vi "shutter_init.vi"(7 "servo":i32(ring)=1 items=["ServoUnspecified", "ServoCh1", "ServoCh2", "ServoBoth"], 8 "error in (no error)":errorcluster, 11 "channel":refnum<k24>) -> (0 "error out":errorcluster)   [LabVIEW 2021]
uses:
  D:/VEP/lib/Grpc.Core.dll
  lib/Grpc.Core.dll
  D:/VEP/lib/FossilProtosSharp.dll
  lib/FossilProtosSharp.dll
panel:
  out "Servo2OriginState":i32(ring) items=["OriginUnspecified", "OriginOk", "OriginGoToEndPlus", "OriginGoToEndMinus", "OriginError", "OriginUnknown"]
  out "Servo1OriginStateFieldNumber":i32
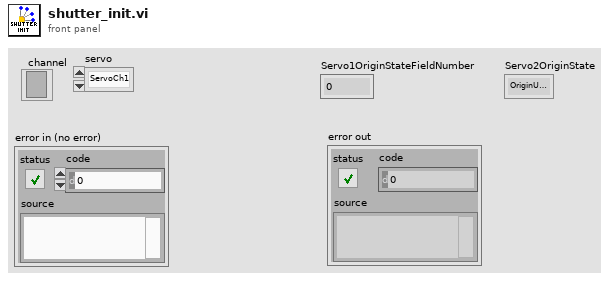
[diagram p1: front panel]
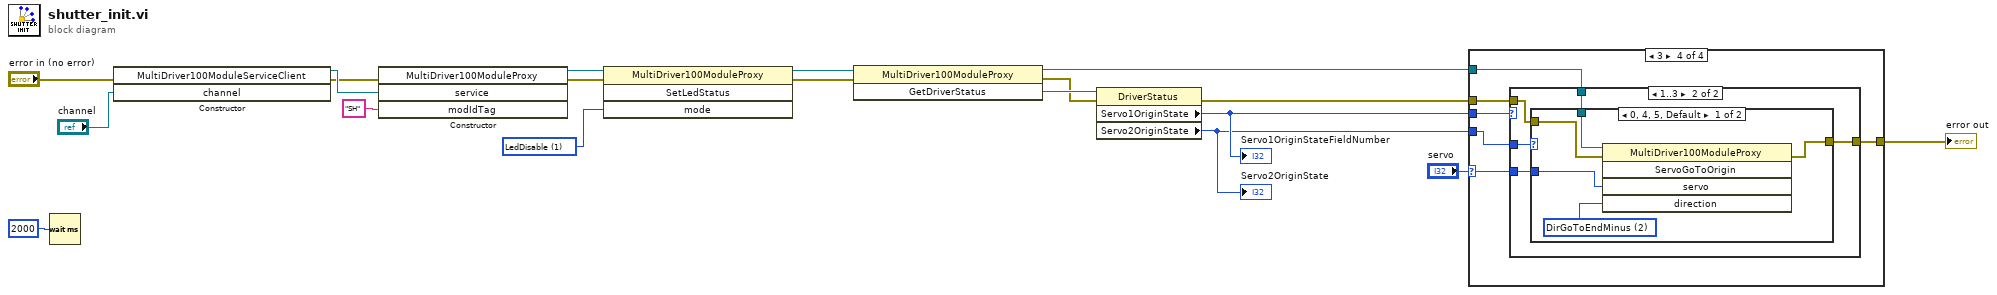
[diagram p0: block diagram]
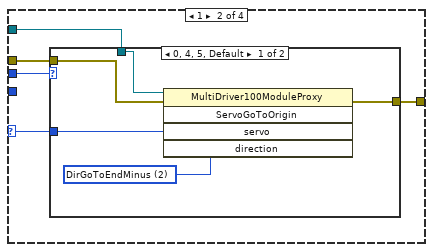
[diagram p3: hidden frame]
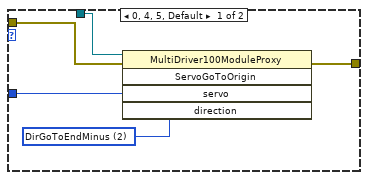
[diagram p6: hidden frame]
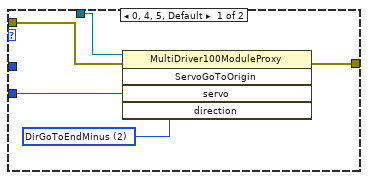
[diagram p7: hidden frame]
diagram:
  w13 = 1 items=["LedUnspecified", "LedDisable", "LedEnable", "LedOnlyErrors", "LedStatus"] ("mode")
  n1 = Wait (ms)(milliseconds to wait=u32 2000) -> ()  [unwired: 1 out]
  n2 = constructor class="MultiDriver100ModuleServiceClie"(error in="error in (no error)", "channel"="channel") -> (reference out=w18:refnum<k24>, error out=w17:errorcluster)  [unwired: 2 in, 2 out]
  n3 = constructor class="MultiDriver100ModuleProxy"(error in=w17, "service"=w18, "modIdTag"="SH") -> (reference out=w14:refnum<k24>, error out=w12:errorcluster)  [unwired: 2 in, 3 out]
  n4 = invoke class="MultiDriver100ModuleProxy" method="SetLedStatus"(reference=w14, error in=w12, "mode"=w13) -> (reference out=w10:refnum<k24>, error out=w8:errorcluster)  [unwired: 1 in, 2 out]
  n5 = invoke class="MultiDriver100ModuleProxy" method="GetDriverStatus"(reference=w10, error in=w8) -> (reference out=w6:refnum<k24>, error out=w5:errorcluster, "GetDriverStatus"=w9:refnum<k24>)  [unwired: 1 in]
  n6 = property class="DriverStatus"(reference=w9, error in=w5) -> (error out=w4:errorcluster, "Servo1OriginState"=w3:i32, "Servo2OriginState"=w2:i32)  [unwired: 1 out]
  "Servo1OriginStateFieldNumber" <- w3
  "Servo2OriginState" <- w2
  n7 = case shown="3" "servo" {
    selector: "servo" -> [_ w22 w34 w45]
    tunnel: w6 -> [_ w24 w36 w47]
    tunnel: w4 -> [w20 w23 w35 w46]
    tunnel: w3 -> [_ w25 _ w48]
    tunnel: w2 -> [_ _ w32 w43]
    tunnel: [w20 w21 w33 w44] -> w1
    frame 0, Default {
      # "servo unspecified - do nothing"
    }
    frame 1 {
      n8 = case shown="0, 4, 5, Default" w25 {
        tunnel: w24 -> [w30 _]
        tunnel: w23 -> [w29 w31]
        tunnel: w22 -> [w28 _]
        tunnel: [w26 w31] -> w21
        frame 0, 4, 5, Default {
          w27 = 2 items=["DirUnspecified", "DirGoToEndPlus", "DirGoToEndMinus"] ("direction")
          n9 = invoke class="MultiDriver100ModuleProxy" method="ServoGoToOrigin"(reference=w30, error in=w29, "servo"=w28, "direction"=w27) -> (error out=w26:errorcluster)  [unwired: 1 in, 4 out]
        }
        frame 1..3 {
          # "Origin specified or about to be specified - do nothing"
        }
      }
    }
    frame 2 {
      n10 = case shown="1..3" w32 {
        tunnel: w36 -> [w41 _]
        tunnel: w35 -> [w40 w42]
        tunnel: w34 -> [w39 _]
        tunnel: [w37 w42] -> w33
        frame 0, 4, 5, Default {
          w38 = 2 items=["DirUnspecified", "DirGoToEndPlus", "DirGoToEndMinus"] ("direction")
          n11 = invoke class="MultiDriver100ModuleProxy" method="ServoGoToOrigin"(reference=w41, error in=w40, "servo"=w39, "direction"=w38) -> (error out=w37:errorcluster)  [unwired: 1 in, 4 out]
        }
        frame 1..3 {
          # "Origin specified or about to be specified - do nothing"
        }
      }
    }
    frame 3 {
      n12 = case shown="1..3" w48 {
        tunnel: w47 -> [w53 w55]
        tunnel: w46 -> [w52 w57]
        tunnel: w45 -> [w51 w54]
        tunnel: [w49 w56] -> w44
        tunnel: w43 -> [_ w58]
        frame 0, 4, 5, Default {
          w50 = 2 items=["DirUnspecified", "DirGoToEndPlus", "DirGoToEndMinus"] ("direction")
          n13 = invoke class="MultiDriver100ModuleProxy" method="ServoGoToOrigin"(reference=w53, error in=w52, "servo"=w51, "direction"=w50) -> (error out=w49:errorcluster)  [unwired: 1 in, 4 out]
        }
        frame 1..3 {
          n14 = case shown="0, 4, 5, Default" w58 {
            tunnel: w57 -> [w62 w64]
            tunnel: [w61 w64] -> w56
            tunnel: w55 -> [w63 _]
            tunnel: w54 -> [w60 _]
            frame 0, 4, 5, Default {
              w59 = 2 items=["DirUnspecified", "DirGoToEndPlus", "DirGoToEndMinus"] ("direction")
              n15 = invoke class="MultiDriver100ModuleProxy" method="ServoGoToOrigin"(reference=w63, error in=w62, "servo"=w60, "direction"=w59) -> (error out=w61:errorcluster)  [unwired: 1 in, 4 out]
            }
            frame 1..3 {
            }
          }
        }
      }
    }
  }
  "error out" <- w1
